vi "Swerve Drive.vi"(0 "X":dbl(slide) scale=-1.0..1.0, 1 "Rot. Point Y":dbl, 3 "Rot. Point X":dbl, 7 "Y":dbl(slide) scale=1.0..-1.0, 11 "Z":dbl(knob) scale=1.0..-1.0, 13 "Robot-Centric":bool) -> ()   [LabVIEW 2018]
panel:
  # "SWERVE DRIVE\nVersion 3.1B\n\nCory Lynch\nApple Pi Robotics\nTeam 2067\n\nAdapted by\nDavid Genois\nfor Team 5443"
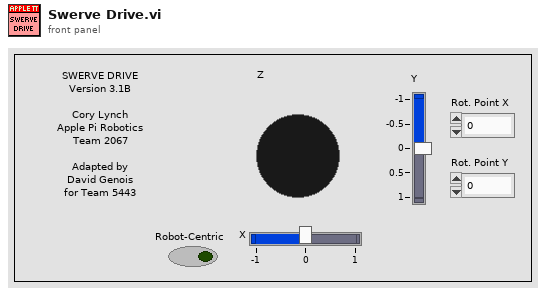
[diagram p1: front panel]
types:
  T1 = enum16{"Back Left", "Back Right", "Front Left", "Front Right"}
  T2 = typedef "WPI_GyroDevRef.ctl" = cluster{"DevStatus":errorcluster, "Analog Channel":T3, "Gain (VoltsPerDegree/Second)":dbl, "Gyro Type":enum16{"Analog", "XRS450"}, "Handle":i32, "SPI Bus":T4, "Device Found":bool, "Sample Rate":dbl, "Calibrate On Open":bool, "Offset":dbl}
  T3 = typedef "FPGA_AIChannel.ctl" = enum8{"AI 0", "AI 1", "AI 2", "AI 3", "AI MXP 0", "AI MXP 1", "AI MXP 2", "AI MXP 3", "Invalid"}
  T4 = typedef "spi_bus.ctl" = enum16{"SPI On-Board, CS0", "SPI On-Board, CS1", "SPI On-Board, CS2", "SPI On-Board, CS3", "SPI MXP", "Invalid"}
  T5 = typedef "WPI_MotorControlDeviceRef.ctl" = cluster{"DeviceStatus":errorcluster, "Type":T6, "PWM":cluster{"PWM Channel":T7, "DeadBand":T8}, "CAN":cluster{"Device Number":u8, "SetOutput VI Ref":variant, "GetOutput VI Ref":variant, "Enable VI Ref":variant, "Disable VI Ref":variant, "Data":variant}, "Invert":bool, "DIO PWM":cluster{"PWM \"Enable\" Channel":T7, "DIOChannel":T9, "PWM Rate":dbl}}
  T6 = typedef "WPI_MotorControlType.ctl" = enum16{"PWM", "CAN", "DIO PWM"}
  T7 = typedef "FPGA_DIOPWMChannel.ctl" = enum8{"PWM 0", "PWM 1", "PWM 2", "PWM 3", "PWM 4", "PWM 5", "PWM 6", "PWM 7", "PWM 8", "PWM 9", "PWM MXP 0", "PWM MXP 1", "PWM MXP 2", "PWM MXP 3", "PWM MXP 4", "PWM MXP 5", "PWM MXP 6", "PWM MXP 7", "PWM MXP 8", "PWM MXP 9", "Invalid"}
  T8 = typedef "WPI_PWMDeadband.ctl" = cluster{"Name":string, "maxPositivePwm":i32, "minPositivePwm":i32, "centerPwm":i32, "maxNegativePwm":i32, "minNegativePwm":i32, "angularRange":u16}
  T9 = typedef "FPGA_DIOChannel.ctl" = enum8{"DIO 0", "DIO 1", "DIO 2", "DIO 3", "DIO 4", "DIO 5", "DIO 6", "DIO 7", "DIO 8", "DIO 9", "DIO MXP 0", "DIO MXP 1", "DIO MXP 2", "DIO MXP 3", "DIO MXP 4", "DIO MXP 5", "DIO MXP 6", "DIO MXP 7", "DIO MXP 8", "DIO MXP 9", "DIO MXP 10", "DIO MXP 11", "DIO MXP 12", "DIO MXP 13", "DIO MXP 14", "DIO MXP 15", "SPI Port CS1", "SPI Port CS2", "SPI Port CS3", "SPI Port MISO", "SPI Port MOSI", "Invalid"}
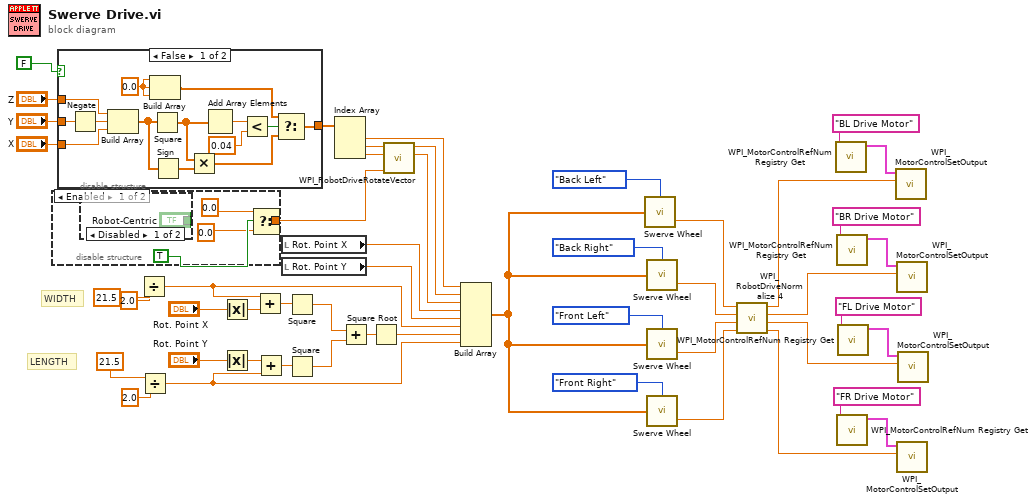
[diagram p0: block diagram]
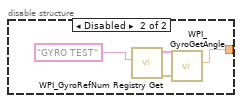
[diagram p3: hidden frame]
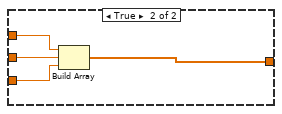
[diagram p4: hidden frame]
diagram:
  # "LENGTH"
  # "WIDTH"
  n1 = disable-structure shown="Enabled" {
    disable-tunnel: [w53 w59] -> w4
    frame Enabled {
      n2 = disable-structure shown="Disabled" {
        disable-tunnel: ["Robot-Centric" _] -> _
        frame Disabled {
        }
        frame Enabled {
        }
      }
      n3 = Select(t=0.0, s=TRUE, f=0.0) -> (s? t:f=w53:dbl)
    }
    frame Disabled {
      n4 = call <vilib>:"WPI_GyroRefNum Registry Get.vi"("refnum name"="GYRO TEST") -> ("error out"=w58:errorcluster, "GyroDevRef"=w57:T2)  [unwired: 9 in]
      n5 = call <vilib>:"WPI_GyroGetAngle.vi"("error in"=w58, "GyroDevRef"=w57) -> ("Angle"=w59:dbl)  [unwired: 5 in, 4 out]
    }
  }
  n6 = case shown="False" FALSE {
    tunnel: "Y" -> [w70 w76]
    tunnel: "X" -> [w64 w77]
    tunnel: "Z" -> [w60 w74]
    tunnel: [w61 w75] -> w7
    frame False {
      w68 = 0.0 ("element")
      n7 = Negate(x=w70) -> (-x=w63:dbl)
      n8 = Build Array(w60, w63, w64) -> (w67:dbl[])
      n9 = Build Array(w68, w68, w68) -> (w69:dbl[])
      n10 = Square(x=w67) -> (x^2=w65:dbl[])
      n11 = Sign(1:w67) -> (0:w66:dbl[])
      n12 = Multiply(x=w65, y=w66) -> (x*y=w62:dbl[])
      n13 = Add Array Elements(numeric array=w65) -> (sum=w73:dbl)
      n14 = Less?(x=w73, y=0.04 ("x")) -> (x < y?=w71:bool)
      n15 = Select(t=w69, s=w71, f=w62) -> (s? t:f=w61:dbl[])
    }
    frame True {
      n16 = Build Array(w74, w76, w77) -> (w75:dbl[])
    }
  }
  n17 = Divide(x=21.5 ("Robot Width"), y=2.0) -> (x/y=w11:dbl)
  n18 = Divide(x=21.5 ("Robot Length"), y=2.0) -> (x/y=w9:dbl)
  n19 = Absolute Value(x="Rot. Point X") -> (abs(x)=w29:dbl)
  n20 = Absolute Value(x="Rot. Point Y") -> (abs(x)=w27:dbl)
  n21 = Add(x=w11, y=w29) -> (x+y=w28:dbl)
  n22 = Add(x=w27, y=w9) -> (x+y=w26:dbl)
  n23 = local read "Rot. Point X"() -> (w13:dbl)
  n24 = local read "Rot. Point Y"() -> (w12:dbl)
  n25 = Square(x=w28) -> (x^2=w24:dbl)
  n26 = Square(x=w26) -> (x^2=w25:dbl)
  n27 = Index Array(array=w7) -> (element #1=w3:dbl, element #2=w8:dbl, element #3=w16:dbl)  [unwired: 3 in]
  n28 = Add(x=w24, y=w25) -> (x+y=w23:dbl)
  n29 = Square Root(x=w23) -> (sqrt(x)=w10:dbl)
  n30 = call <vilib>:"WPI_RobotDriveRotateVector.vi"("Angle"=w4, "X"=w16, "Y"=w8) -> ("X'"=w5:dbl, "Y'"=w2:dbl)  [unwired: 7 out]
  n31 = Build Array(w3, w2, w5, w13, w12, w11, w10, w9) -> (w6:dbl[])
  n32 = call "Swerve Wheel.vi"("Wheel"=T1."Back Left", "Inputs"=w6) -> ("Speed"=w47:dbl)  [unwired: 3 in]
  n33 = call "Swerve Wheel.vi"("Wheel"=T1."Back Right", "Inputs"=w6) -> ("Speed"=w46:dbl)  [unwired: 3 in]
  n34 = call "Swerve Wheel.vi"("Wheel"=T1."Front Left", "Inputs"=w6) -> ("Speed"=w45:dbl)  [unwired: 3 in]
  n35 = call "Swerve Wheel.vi"("Wheel"=T1."Front Right", "Inputs"=w6) -> ("Speed"=w44:dbl)  [unwired: 3 in]
  n36 = call <vilib>:"WPI_RobotDriveNormalize 4.vi"("D"=w44, "C"=w45, "B"=w46, "A"=w47) -> ("D'"=w31:dbl, "C'"=w32:dbl, "B'"=w33:dbl, "A'"=w34:dbl)
  n37 = call <vilib>:"WPI_MotorControlRefNum Registry Get.vi"("refnum name"="BL Drive Motor") -> ("MotorControlDevRef"=w42:T5)  [unwired: 9 in, 1 out]
  n38 = call <vilib>:"WPI_MotorControlRefNum Registry Get.vi"("refnum name"="BR Drive Motor") -> ("MotorControlDevRef"=w39:T5)  [unwired: 9 in, 1 out]
  n39 = call <vilib>:"WPI_MotorControlRefNum Registry Get.vi"("refnum name"="FR Drive Motor") -> ("MotorControlDevRef"=w35:T5)  [unwired: 9 in, 1 out]
  n40 = call <vilib>:"WPI_MotorControlRefNum Registry Get.vi"("refnum name"="FL Drive Motor") -> ("MotorControlDevRef"=w38:T5)  [unwired: 9 in, 1 out]
  n41 = call <vilib>:"WPI_MotorControlSetOutput.vi"("Output"=w34, "MotorControlDevRef"=w42) -> ()  [unwired: 7 in, 3 out]
  n42 = call <vilib>:"WPI_MotorControlSetOutput.vi"("Output"=w33, "MotorControlDevRef"=w39) -> ()  [unwired: 7 in, 3 out]
  n43 = call <vilib>:"WPI_MotorControlSetOutput.vi"("Output"=w31, "MotorControlDevRef"=w35) -> ()  [unwired: 7 in, 3 out]
  n44 = call <vilib>:"WPI_MotorControlSetOutput.vi"("Output"=w32, "MotorControlDevRef"=w38) -> ()  [unwired: 7 in, 3 out]
